vi "XNode Template Single.vi"(0 "failure in":T1 {"code" format="%.0x"}, 1 "Tag":string, 5 "Value":variant) -> (4 "failure out":T1 {"code" format="%.0x"}, 8 "failed":bool)   [LabVIEW 2013, in "Write Exception Property.xnode"]
doc: "This VI is used to store data similar to a look up table, into a Variant data type. This VI is will set an attribute of the <b>Variant Repository In</b>, with the tag name of <b>Tag</b>, value of <b>Value</b>, and then return the new <b>Varient Repository Out</b>. This VI will also return whether or not the new tag being written is replacing an old one or not, in the <b>Replaced?</b> boolean.\n\nThe tag name it self is optional and if one is not provided then the label name on the <b>Value</b> data will be used.\n\nOptionally the <b>Write Once?</b> boolean can be used. If true this will generate an error, if the tag that is trying to be written is already written. In this way the tag can only be written once without generating an error. By default this is set to false.\n\nTo read multiple tags right click and choose Read Multiple Tags.\n\n-------------\nBrian Hoover (Hooovahh)\n\nProduct Name: Variant Repository\nPackage File Name: lava_lib_variant_repository\nPackage Version: 1.0.1.11\nMinimum LabVIEW Version: 11.0"
uses:
  Write Exception Property.xnode
  failure.ctl
  <vilib>/Utility/VariantDataType/VariantType.lvlib
  failure.lvlib
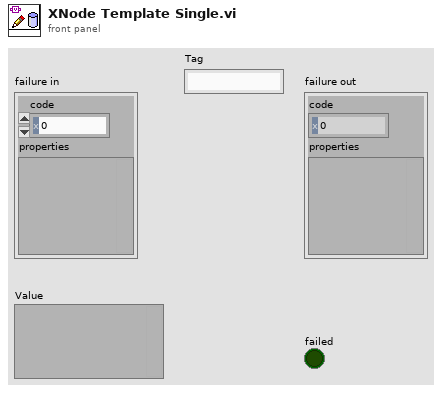
[diagram p1: front panel]
types:
  T1 = typedef "failure.lvlib/failure.ctl" = cluster{"code":i32, "properties":variant}
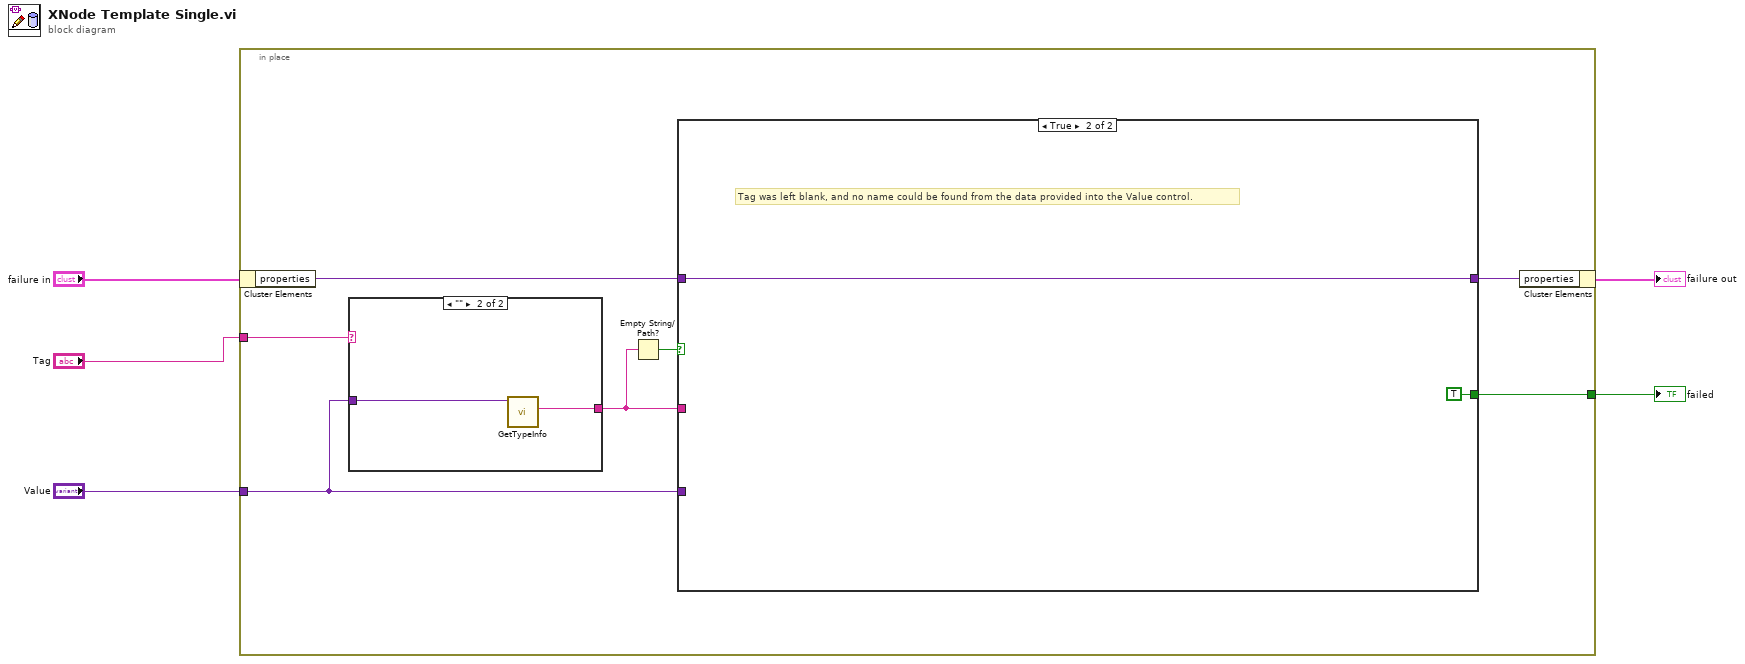
[diagram p0: block diagram]
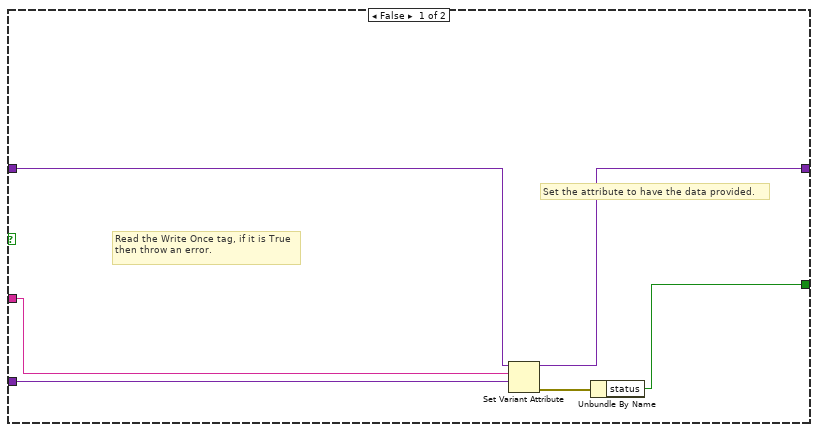
[diagram p2: hidden frame]
diagram:
  n1 = in-place {
    in-place-border: "Tag" -> [w12]
    in-place-border: "Value" -> [w11]
    in-place-border: [w8] -> w2
    n2 = in-place-cluster #1("failure in") -> ("properties"=w10:variant)
    n3 = case shown="\"\"" w12 {
      selector: w12 -> [w21 _]
      tunnel: [w21 w23] -> w7
      tunnel: w11 -> [_ w22]
      frame Default {
      }
      frame "" {
        n4 = call <vilib>:"GetTypeInfo.vi"("Variant"=w22) -> ("Name"=w23:string)  [unwired: 6 in, 4 out]
      }
    }
    n5 = Empty String/Path?(string/path=w7) -> (empty?=w6:bool)
    n6 = case shown="True" w6 {
      tunnel: [w18 w20] -> w9
      tunnel: w10 -> [w15 w20]
      tunnel: w11 -> [w17 _]
      tunnel: w7 -> [w14 _]
      tunnel: [w16 TRUE ("status")] -> w8
      frame False {
        # "Set the attribute to have the data provided."
        # "Read the Write Once tag, if it is True then throw an error."
        n7 = Set Variant Attribute(Variant=w15, name=w14, value=w17) -> (Variant out=w18:variant, error out=w13:errorcluster)  [unwired: 1 in, 1 out]
        n8 = Unbundle By Name(w13) -> ("status"=w16:bool)
      }
      frame True {
        # "Tag was left blank, and no name could be found from the data provided into the Value control."
      }
    }
    n9 = in-place-cluster #1("properties"=w9) -> (→"failure out":T1)
  }
  "failed" <- w2
